vi "Prompt for Power On.vi"(8 "Error in":errorcluster caption="Error in (no error)") -> (0 "Error out":errorcluster, 3 "Pass":bool)   [LabVIEW 2015, in "Rocom Connect.lvclass"]
uses:
  Rocom Connect/Rocom Connect.lvclass
panel:
  in  "Pass":bool=TRUE
  # "Device Turn On"
  # "Connect power to the Wall\nControl Dimmer and press Done"
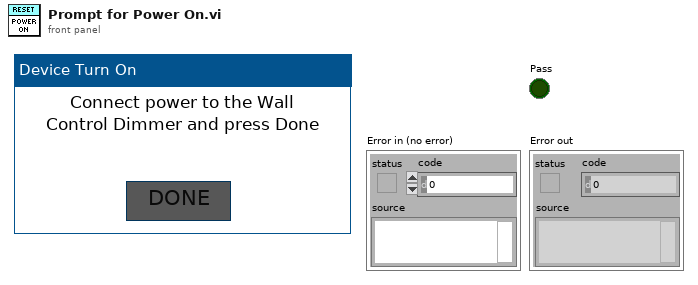
[diagram p1: front panel]
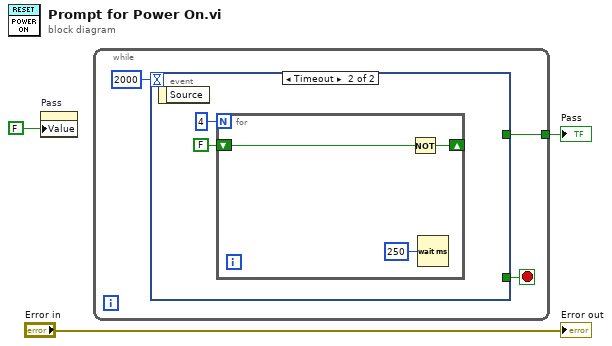
[diagram p0: block diagram]
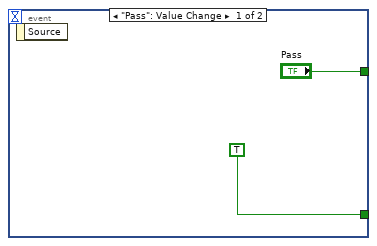
[diagram p2: hidden frame]
diagram:
  n1 = property on="Pass" class="Bool (strict)"("Value"=FALSE ("LED State")) -> ()  [unwired: 2 in, 2 out]
  n2 = while {
    tunnel: [w6] -> w3
    stop <- w5 stop-if-true
    n3 = event shown="[1] Timeout" {
      selector: _ -> [_ _]
      dyn-events: _ -> [_ _]
      timeout: 2000 -> [_ _]
      tunnel: ["Pass" _] -> w6
      tunnel: [TRUE _] -> w5
      event "Pass": Value Change {
        n4 = event-data() -> ()  [unwired: 1 in, 1 out]
      }
      event Timeout {
        n5 = event-data() -> ()  [unwired: 1 in, 1 out]
        n6 = for {
          N: 4 -> [_]
          shift-right: [w13] -> _
          shift-left: FALSE ("LED State") -> [w11]
          n7 = Not(x=w11) -> (.not. x?=w13:bool)
          n8 = Wait (ms)(milliseconds to wait=u32 250) -> ()  [unwired: 1 out]
        }
      }
    }
  }
  "Pass" <- w3
  "Error out" <- "Error in"
